vi "write_into_db.vi"(7 "Array":string[](array[string]), 8 "Data":variant, 9 "Columns":string[](array[string]), 10 "Table":string, 11 "connection information":path) -> ()   [LabVIEW 2017]
uses:
  6fbb3a4f-da49-41fb-a2a6-52bdda07043b.vi
  <vilib>/addons/database/Connection.llb/DB Tools Open Connec (Path).vi
  <vilib>/addons/database/NI_Database_API.lvlib
panel:
  # "This VI insert Data from an Array into a specific table and columns of a DataBase\n\n1. Choose the UDL connection file for the proper DataBase\n2. Set the desired Table Name and Columns\n3. Write the Data to insert into the DataBase in the Array.\n4. Run this VI"
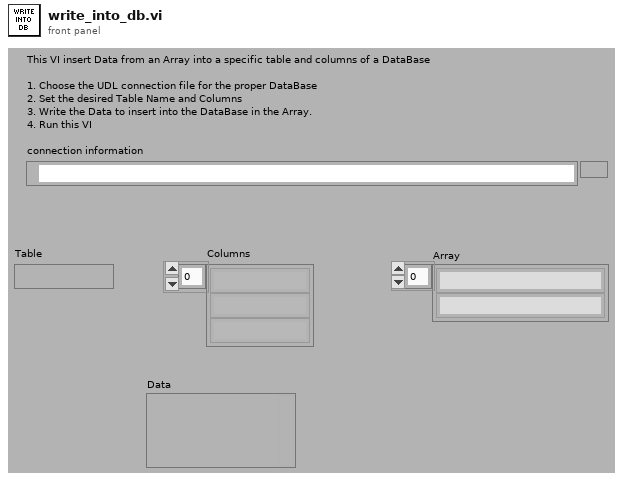
[diagram p1: front panel]
types:
  T1 = cluster{"Temperature":string, "Humidity":string, "Timestamp":string}
  T2 = typedef "NI_Database_API.lvlib/Conn ObjectReference.ctl" = refnum<k1>
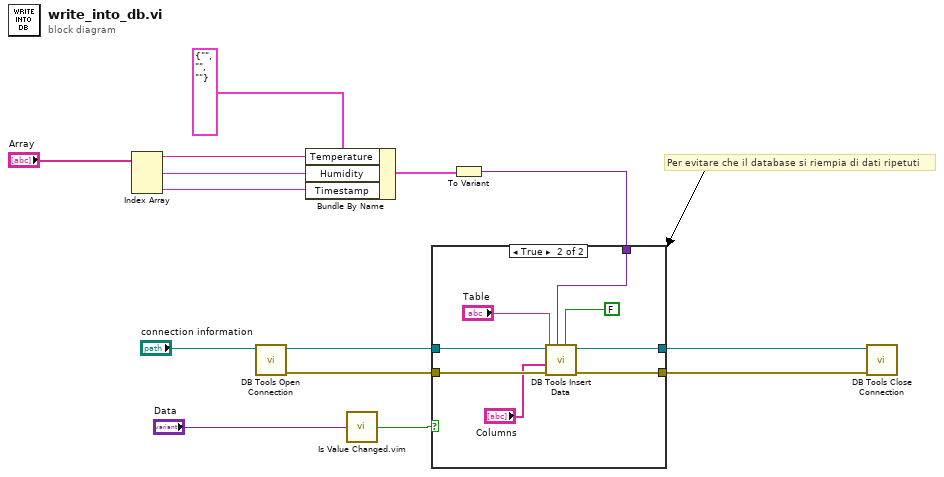
[diagram p0: block diagram]
diagram:
  # "Per evitare che il database si riempia di dati ripetuti"
  n1 = Index Array(array="Array") -> (element #1=w6:string, element #2=w5:string, element #3=w3:string)  [unwired: 3 in]
  n2 = call-poly <vilib>:"DB Tools Open Connection.vi"("connection information"="connection information") -> ("error out"=w11:errorcluster, "connection reference"=w12:T2)  [unwired: 4 in, 3 out]
  n3 = Bundle By Name(cluster=T1 {"Temperature"="", "Humidity"="", "Timestamp"=""}, "Temperature"=w6, "Humidity"=w5, "Timestamp"=w3) -> (w4:T1)
  n4 = call "Is Value Changed.vim"("value"="Data") -> ("changed or first call?"=w1:bool)
  n5 = To Variant(anything=w4) -> (Variant=w8:variant)
  n6 = case shown="True" w1 {
    tunnel: w12 -> [w16 w24]
    tunnel: w11 -> [w15 w23]
    tunnel: [w16 w21] -> w10
    tunnel: [w15 w20] -> w9
    tunnel: w8 -> [_ w19]
    frame False {
    }
    frame True {
      n7 = call <vilib>:"DB Tools Insert Data.vi"("create table? (F)"=FALSE ("create table? (f)"), "data"=w19, "error in (no error)"=w23, "columns"="Columns", "table"="Table", "connection reference"=w24) -> ("error out"=w20:errorcluster, "connection reference out"=w21:T2)  [unwired: 1 in, 3 out]
    }
  }
  n8 = call <vilib>:"DB Tools Close Connection.vi"("error in (no error)"=w9, "connection reference"=w10) -> ()  [unwired: 6 out]
